vi "Initialize Sift Flow.vi"(7 "API URL":string, 9 "API Key":string, 11 "Run Name":string) -> ()   [LabVIEW 2024, in "StreamWriter.lvlib" / "StreamWriter.lvclass"]
uses:
  StreamWriter.lvclass
  StreamWriter.lvclass/StreamWriter.ctl
  src/Sift/Sift API/Sift Client.lvclass
  src/Sift/Sift API/Types/Data Type.ctl
  src/Sift/Sift Client.lvlib
  <vilib>/FlexLogger/SDK/PluginSDK.lvlibp/PEFClasses/SDK/Plugin/Plugin.lvclass
panel:
  in  "Plugin in":refnum<class "StreamWriter.lvclass">
  in  "error in":errorcluster
  out "Sift Client out":refnum<class "Sift Client.lvclass">
  out "error out":errorcluster
  out "Run URL":string
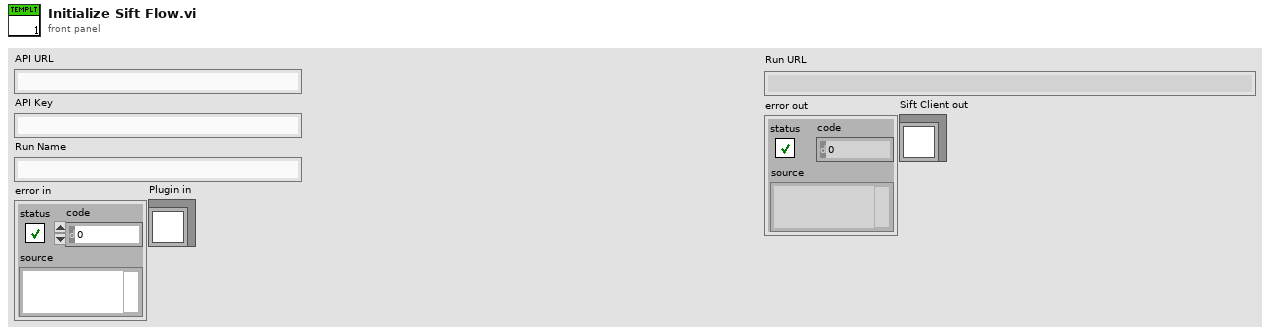
[diagram p1: front panel]
types:
  T1 = typedef "Sift Client.lvlib/Data Type.ctl" = enum8{"double", "float", "uint64", "int64", "uint32", "int32", "bool", "enum", "string"}
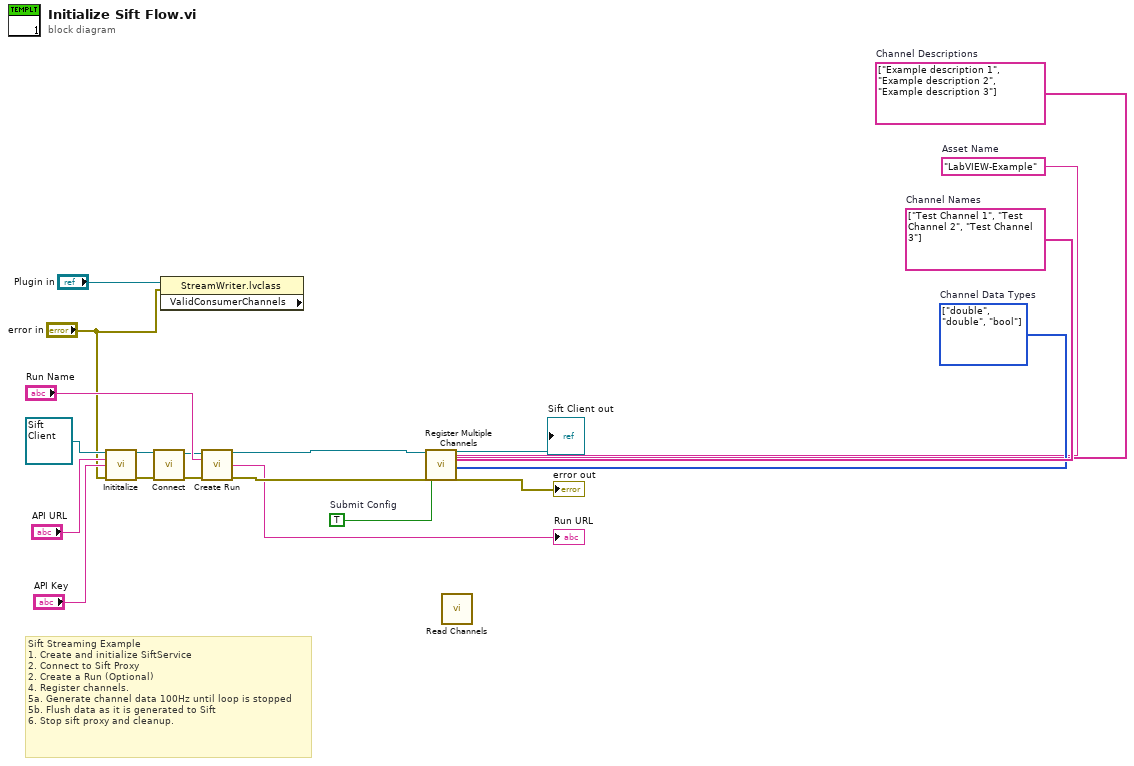
[diagram p0: block diagram]
diagram:
  w10 = TRUE  # Submit Config
  w13 = "LabVIEW-Example"  # Asset Name
  w15 = T1[] [enum."double", enum."double", enum."bool"] items=["double", "float", "uint64", "int64", "uint32", "int32", "bool", "enum", "string"]  # Channel Data Types
  w14 = string[] ["Example description 1", "Example description 2", "Example description 3"]  # Channel Descriptions
  w16 = string[] ["Test Channel 1", "Test Channel 2", "Test Channel 3"]  # Channel Names
  # "Sift Streaming Example\n1. Create and initialize SiftService\n2. Connect to Sift Proxy\n2. Create a Run (Optional)\n4. Register channels.\n5a. Generate channel data 100Hz until loop is stopped\n5b. Flush data as it is generated to Sift\n6. Stop sift proxy and cleanup."
  n1 = call-dynamic "Inititalize.vi"("Sift Client in"=refnum<class "Sift Client.lvclass"> refnum ("Sift Client.lvlib:Sift Client.lvclass"), "API URL"="API URL", "API Key"="API Key", "error in (no error)"="error in") -> ("Sift Client out"=w9:refnum<class "Sift Client.lvclass">, "error out"=w7:errorcluster)  [unwired: 10 in]
  n2 = call-dynamic "Connect.vi"("error in (no error)"=w7, "Sift Client in"=w9) -> ("error out"=w6:errorcluster, "Sift Client out"=w8:refnum<class "Sift Client.lvclass">)  [unwired: 7 in, 1 out]
  n3 = property class="StreamWriter.lvclass" props=["ValidConsumerChannels"](reference="Plugin in", error in="error in") -> ()  [unwired: 3 out]
  n4 = call-dynamic "Create Run.vi"("Sift Client in"=w8, "Name"="Run Name", "error in (no error)"=w6) -> ("Sift Client out"=w11:refnum<class "Sift Client.lvclass">, "URL"=→"Run URL":string, "error out"=w12:errorcluster)  [unwired: 9 in, 1 out]
  n5 = call "Register Multiple Channels.vi"("Sift Client in"=w11, "Asset Name"=w13, "Names"=w16, "Data Types"=w15, "error in (no error)"=w12, "Submit Config"=w10, "Descriptions"=w14) -> ("Sift Client out"=→"Sift Client out":refnum<class "Sift Client.lvclass">, "error out"=→"error out":errorcluster)  [unwired: 19 in]
  n6 = call <vilib>:"Read Channels.vi"() -> ()  [unwired: 9 in, 3 out]
